vi "Append Array Element.vi"(8 "error in (no error)":errorcluster, 9 "JSON Value in":refnum<class "JSON Value.lvclass">, 11 "JSON Value in":refnum<class "JSON Value.lvclass">) -> (0 "error out":errorcluster, 2 "JSON Value out":refnum<class "JSON Value.lvclass">)   [LabVIEW 2017, in "JSON Value.lvclass"]
doc: "Appends an array element to an existing JSON Array"
uses:
  JSON Value.lvclass
  JSON Value.lvclass/JSON Value.ctl
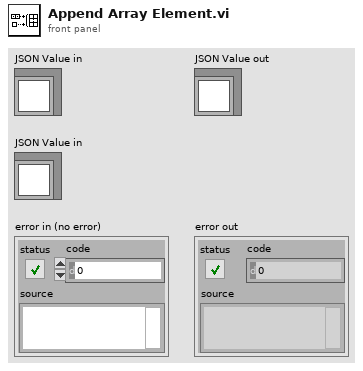
[diagram p1: front panel]
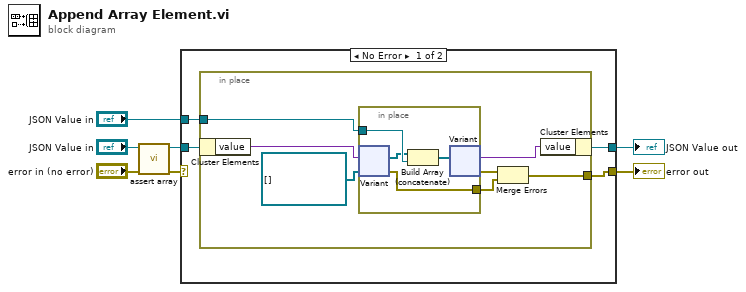
[diagram p0: block diagram]
diagram:
  n1 = call "assert array.vi"("error in (no error)"="error in (no error)", "JSON Value in"="JSON Value in") -> ("error out"=w4:errorcluster, "JSON Value out"=w2:refnum<class "JSON Value.lvclass">)  [unwired: 8 in]
  n2 = case shown="No Error" w4 {
    selector: w4 -> [_ w23]
    tunnel: w2 -> [w11 w24]
    tunnel: [w10 w24] -> w7
    tunnel: "JSON Value in" -> [w9 _]
    tunnel: [w8 w23] -> w1
    frame No Error {
      n3 = in-place {
        in-place-border: w9 -> [w18]
        in-place-border: [w12] -> w8
        n4 = in-place-cluster #1(w11) -> ("value"=w17:variant)
        n5 = in-place {
          in-place-border: w18 -> [w22]
          in-place-border: [w19] -> w13
          n6 = in-place-variant #2(w17, refnum<class "JSON Value.lvclass">[] [] ("JSON Array in")) -> (w21:refnum<class "JSON Value.lvclass">[], w19:errorcluster)
          n7 = Build Array (concatenate)(w21, w22) -> (w20:refnum<class "JSON Value.lvclass">[])
          n8 = in-place-variant #2(w20) -> (w15:variant, w14:errorcluster)
        }
        n9 = Merge Errors(w14, w13) -> (w12:errorcluster)
        n10 = in-place-cluster #1("value"=w15) -> (w10:refnum<class "JSON Value.lvclass">)
      }
    }
    frame Error {
    }
  }
  "JSON Value out" <- w7
  "error out" <- w1
